vi "手柄.vi"() -> ()   [LabVIEW 2017]
uses:
  <vilib>/Platform/TimedLoop/XDataNode/timing_clust.ctl
  <vilib>/Platform/TimedLoop/XDataNode/nitl_modes.ctl
  <vilib>/Platform/TimedLoop/XDataNode/wakeup.ctl
  <vilib>/Utility/inputDevices.llb/joystickAcquire.vi
  <vilib>/Platform/TimedLoop/XDataNode/XDataNode.xnode
  <vilib>/Platform/TimedLoop/XDataNode/XDNodeRunTimeDep.lvlib
panel:
  out "axis info":T1 caption="坐标轴信息"
  out "direction info":T2 caption="方向信息"
  out "button info":T3 caption="按钮信息"
  in  "停止":bool
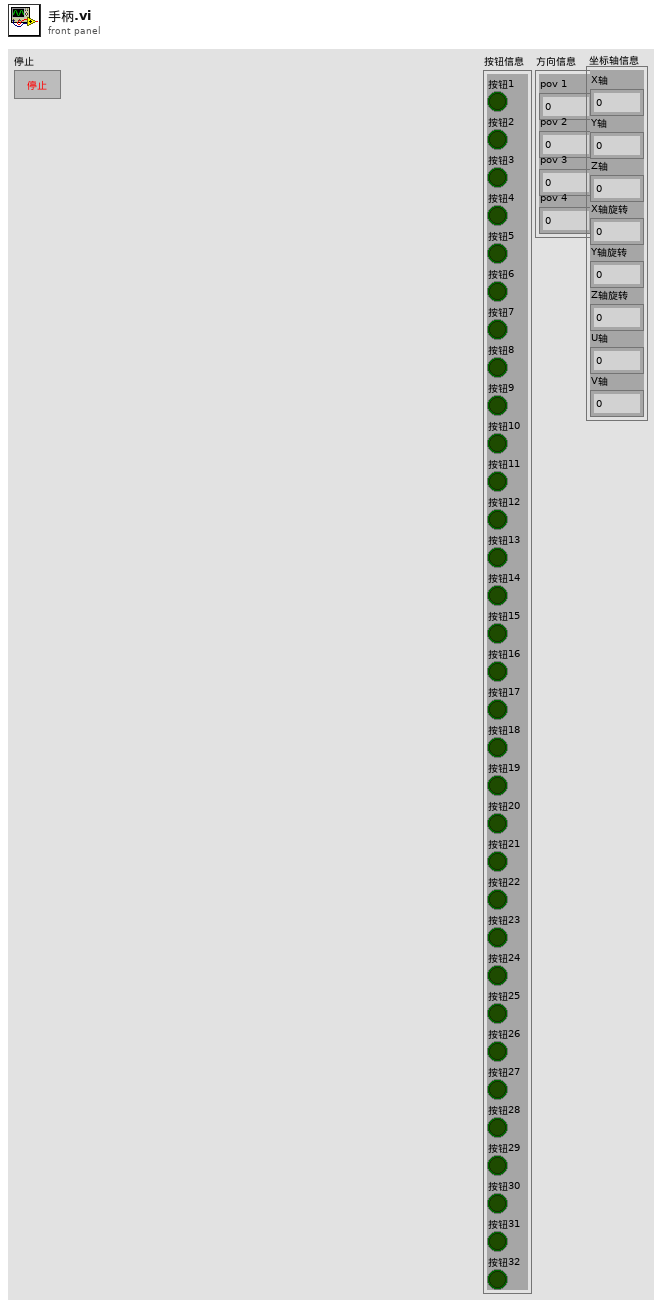
[diagram p1: front panel]
types:
  T1 = cluster{"X axis":i32, "Y axis":i32, "Z axis":i32, "X axis rotation":i32, "Y axis rotation":i32, "Z axis rotation":i32, "U axis":i32, "V axis":i32}
  T2 = cluster{"pov 1":i32, "pov 2":i32, "pov 3":i32, "pov 4":i32}
  T3 = cluster{"button 1":bool, "button 2":bool, "button 3":bool, "button 4":bool, "button 5":bool, "button 6":bool, "button 7":bool, "button 8":bool, "button 9":bool, "button 10":bool, "button 11":bool, "button 12":bool, "button 13":bool, "button 14":bool, "button 15":bool, "button 16":bool, "button 17":bool, "button 18":bool, "button 19":bool, "button 20":bool, "button 21":bool, "button 22":bool, "button 23":bool, "button 24":bool, "button 25":bool, "button 26":bool, "button 27":bool, "button 28":bool, "button 29":bool, "button 30":bool, "button 31":bool, "button 32":bool}
  T4 = cluster{"axes total":u32, "buttons total":u32, "pov total":u32, "device name":string}[]
  T5 = typedef "XDNodeRunTimeDep.lvlib/timing_clust.ctl" = cluster{"Expected End [f-1]":u64, "Actual End [f-1]":u64, "Finished Late? [f-1]":bool, "Expected End [i-1]":u64, "Actual End [i-1]":u64, "Finished Late? [i-1]":bool, "Expected Start [i]":u64, "Actual Start [i]":u64, "Expected Start [f]":u64, "Actual Start [f]":u64, "Source Name":string, "Structure Name":string, "Period":i64, "Deadline":i64, "Offset":i64, "Start":i64, "Priority":i32, "Timeout":i32, "Mode":T6, "Wakeup Reason":T7, "Error":errorcluster, "Source Type":string, "Secondary Source Type":string, "Global End Time":u64, "Global Start Time":u64, "Frame Duration":u64, "Iteration Duration":u64, "Assigned CPU":i32, "I/O Scan Engine Mode":u32}
  T6 = typedef "XDNodeRunTimeDep.lvlib/nitl_modes.ctl" = enum32{"No Change", "Process missed periods, maintain original phase", "Discard missed periods, maintain original phase", "Process missed periods, ignore original phase", "Discard missed periods, ignore original phase"}
  T7 = typedef "XDNodeRunTimeDep.lvlib/wakeup.ctl" = enum32{"Normal", "Aborted", "Asynchronous wakeup", "Timing source error", "Timed loop error", "Timeout"}
  T8 = cluster{"X axis":dbl, "Y axis":dbl, "Z axis":dbl, "X axis rotation":dbl, "Y axis rotation":dbl, "Z axis rotation":dbl, "U axis":dbl, "V axis":dbl}
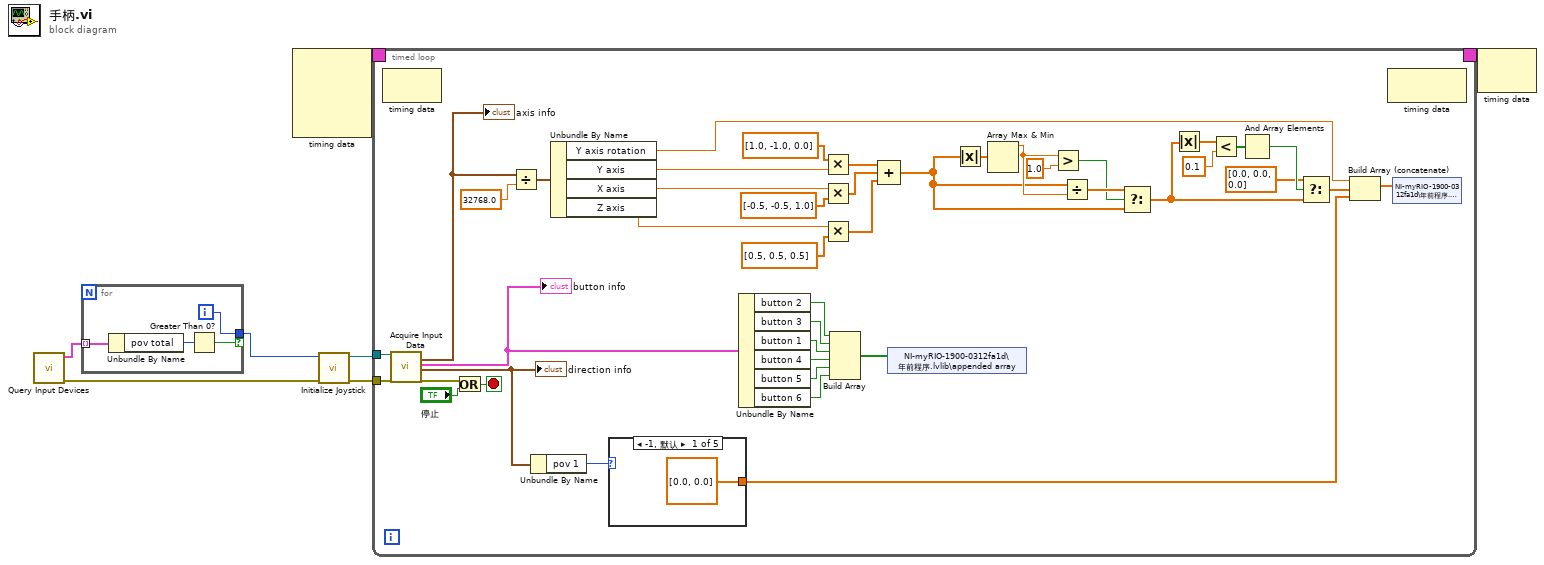
[diagram p0: block diagram]
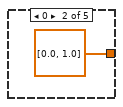
[diagram p2: hidden frame]
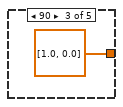
[diagram p3: hidden frame]
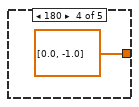
[diagram p4: hidden frame]
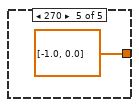
[diagram p5: hidden frame]
diagram:
  n1 = call <vilib>:"Query Input Devices.vi"() -> ("error out"=w5:errorcluster, "joystick info"=w2:T4)  [unwired: 8 in, 2 out]
  n2 = for {
    tunnel: w2 -> [w10] mode=indexing
    tunnel: [w9] -> w1 if=w8
    i -> [w9]
    n3 = Unbundle By Name(w10) -> ("pov total"=w11:u32)
    n4 = Greater Than 0?(x=w11) -> (x > 0?=w8:bool)
  }
  n5 = node-c288() -> (w7:T5)  [unwired: 4 in]
  n6 = call <vilib>:"Initialize Joystick.vi"("error in (no error)"=w5, "device index"=w1) -> ("error out"=w4:errorcluster, "device ID"=w3:refnum<k1>)  [unwired: 8 in]
  n7 = timed-loop {
    timing: w7 -> [_]
    timing-out: [_] -> w6
    tunnel: w4 -> [w54]
    tunnel: w3 -> [w53]
    stop <- w14 stop-if-true
    n8 = node-c288() -> ()  [unwired: 1 in, 1 out]
    n9 = call-poly <vilib>:"Acquire Input Data.vi"("device ID"=w53, "error in (no error)"=w54) -> ("axis info"=w41:T1, "button info"=w27:T3, "direction info"=w17:T2, "error out"=w13:errorcluster)  [unwired: 13 in, 1 out]
    "button info" <- w27
    "direction info" <- w17
    "axis info" <- w41
    n10 = Or(x=w13, y="停止") -> (x .or. y?=w14:bool)
    n11 = Divide(x=w41, y=32768.0) -> (x/y=w39:T8)
    n12 = Unbundle By Name(w17) -> ("pov 1"=w16:i32)
    n13 = Unbundle By Name(w39) -> ("Y axis rotation"=w18:dbl, "Y axis"=w50:dbl, "X axis"=w52:dbl, "Z axis"=w28:dbl)
    n14 = case shown="-1, 默认" w16 {
      tunnel: [dbl[] [0.0, 0.0] dbl[] [0.0, 1.0] dbl[] [1.0, 0.0] dbl[] [0.0, -1.0] dbl[] [-1.0, 0.0]] -> w15
      frame -1, Default {
      }
      frame 0 {
      }
      frame 90 {
      }
      frame 180 {
      }
      frame 270 {
      }
    }
    n15 = Unbundle By Name(w27) -> ("button 2"=w26:bool, "button 3"=w25:bool, "button 1"=w24:bool, "button 4"=w23:bool, "button 5"=w21:bool, "button 6"=w20:bool)
    n16 = Multiply(x=dbl[] [1.0, -1.0, 0.0], y=w50) -> (x*y=w48:dbl[])
    n17 = Multiply(x=w52, y=dbl[] [-0.5, -0.5, 1.0]) -> (x*y=w31:dbl[])
    n18 = Multiply(x=w28, y=dbl[] [0.5, 0.5, 0.5]) -> (x*y=w30:dbl[])
    n19 = Build Array(w26, w25, w24, w23, w21, w20) -> (w22:bool[])
    n20 = Compound Arithmetic op=ADD(w48, w31, w30) -> (w42:dbl[])
    n21 = shared-variable "NI-myRIO-1900-0312fa1d\\年前程序.lvlib\\appended array"(w22) -> ()  [unwired: 1 in, 1 out]
    n22 = Absolute Value(x=w42) -> (abs(x)=w47:dbl[])
    n23 = Array Max & Min(array=w47) -> (max value=w45:dbl)  [unwired: 3 out]
    n24 = Greater?(x=w45, y=1.0) -> (0:w43:bool)
    n25 = Divide(x=w42, y=w45) -> (x/y=w44:dbl[])
    n26 = Select(t=w44, s=w43, f=w42) -> (s? t:f=w35:dbl[])
    n27 = Absolute Value(x=w35) -> (abs(x)=w38:dbl[])
    n28 = Less?(x=w38, y=0.1) -> (x < y?=w36:bool[])
    n29 = And Array Elements(Boolean array=w36) -> (logical AND=w33:bool)
    n30 = Select(t=dbl[] [0.0, 0.0, 0.0], s=w33, f=w35) -> (s? t:f=w34:dbl[])
    n31 = Build Array (concatenate)(w18, w34, w15) -> (w19:dbl[])
    n32 = node-c288() -> ()  [unwired: 1 in, 1 out]
    n33 = shared-variable "NI-myRIO-1900-0312fa1d\\年前程序.lvlib\\数组"(w19) -> ()  [unwired: 1 in, 1 out]
  }
  n34 = node-c288(w6) -> ()  [unwired: 1 out]
